vi "FRCts20_Backend_Comment_GET.vi"(6 "Message Attributes":T4, 8 "error in (no error)":errorcluster, 10 "Data":string, 11 "Engine_Refnums":T1) -> (0 "error out":errorcluster)   [LabVIEW 2014, in "FRCts20_Backend_Engine.lvlib"]
doc: "Retrieves all information about a comment, called by the Comment API. Expects a comment index."
uses:
  FRCts20_Backend_Engine.lvlib
  Dependencies/Keyed Array/KeyedArray.ctl
  FRCts20_Backend_EngineRefnums.ctl
  INI_Accessor/FRCts20_Backend_INI Controller.lvclass
  Dependencies/AMC/_SubVIs/TypeDefs/Message Queue.ctl
  Dependencies/AMC/_SubVIs/TypeDefs/Message.ctl
  <vilib>/addons/database/Connection.llb/Conn ObjectReference.ctl
  FRCts20_Backend_FGVOperation.ctl
  FRCts20_Backend_API/FRCts20_Backend_API_Note.ctl
  FRCts20_Backend_API/FRCts20_Backend_API.lvlib
  Dependencies/Keyed Array/Tools_KeyedArray.lvlib
  Dependencies/AMC/AMC.lvlib
  <vilib>/addons/database/NI_Database_API.lvlib
panel:
  # "DEPRICATED"
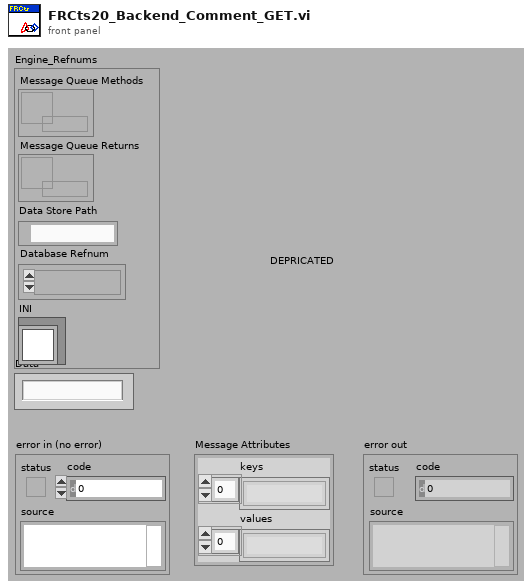
[diagram p1: front panel]
types:
  T1 = typedef "FRCts20_Backend_Engine.lvlib/FRCts20_Backend_EngineRefnums.ctl" = cluster{"Message Queue Methods":T2, "Message Queue Returns":T2, "Data Store Path":path, "Database Refnum":T3, "INI":refnum<class "FRCts20_Backend_INI Controller.lvclass">}
  T2 = typedef "AMC.lvlib/Message Queue.ctl" = refnum<queue>
  T3 = typedef "NI_Database_API.lvlib/Conn ObjectReference.ctl" = refnum<k1>
  T4 = typedef "Tools_KeyedArray.lvlib/KeyedArray.ctl" = cluster{"keys":string[], "values":string[]}
  T5 = typedef "FRCts20_Backend_Engine.lvlib/FRCts20_Backend_API.lvlib/FRCts20_Backend_API_Note.ctl" = cluster{"Note Index":u32, "Request Index":u32, "Author":string, "Time Entered":timestamp, "Text":string, "Solution":bool, "APIReturn":string}
  T6 = typedef "FRCts20_Backend_Engine.lvlib/FRCts20_Backend_FGVOperation.ctl" = enum16{"Initialize", "EnqueueMessage", "EnqueueDataReturn", "FlushMessage", "FlushDataReturn"}
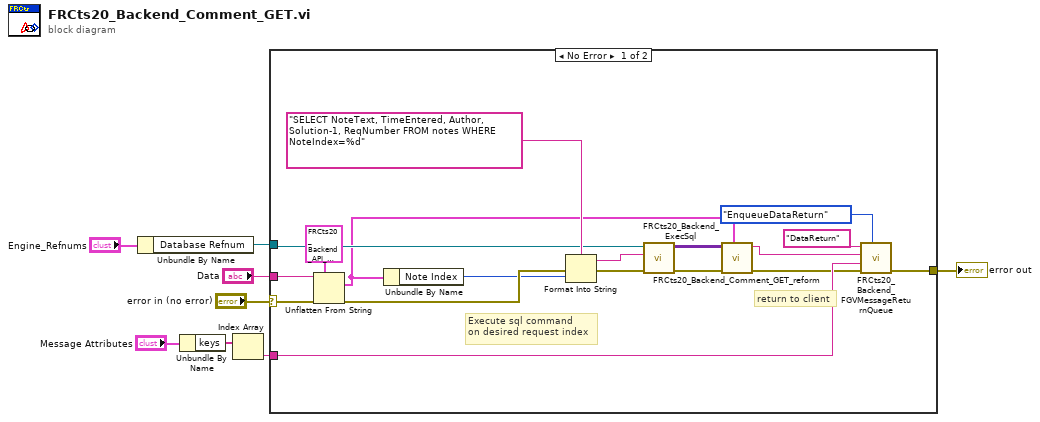
[diagram p0: block diagram]
diagram:
  n1 = Unbundle By Name("Engine_Refnums") -> ("Database Refnum"=w1:T3)
  n2 = Unbundle By Name("Message Attributes") -> ("keys"=w4:string[])
  n3 = Index Array(array=w4) -> (element=w3:string)  [unwired: 1 in]
  n4 = case shown="No Error" "error in (no error)" {
    selector: "error in (no error)" -> [w23 w27]
    tunnel: [w26 w27] -> w7
    tunnel: w1 -> [w14 _]
    tunnel: "Data" -> [w24 _]
    tunnel: w3 -> [w25 _]
    frame No Error {
      # "return to client"
      # "Execute sql command\non desired request index"
      n5 = Unflatten From String(type=T5 {"Note Index"=0, "Request Index"=0, "Author"="", "Time Entered"=timestamp(0 s since 1904-01-01), "Text"="", "Solution"=FALSE, "APIReturn"=""} ("Note"), binary string=w24, error in (no error)=w23) -> (value=w9:T5, error out=w22:errorcluster)  [unwired: 2 in, 1 out]
      n6 = Unbundle By Name(w9) -> ("Note Index"=w20:u32)
      n7 = Format Into String(format string="SELECT NoteText, TimeEntered, Author, Solution-1, ReqNumber FROM notes WHERE NoteIndex=%d", error in=w22, w20) -> (resulting string=w12:string, error out=w13:errorcluster)  [unwired: 1 in]
      n8 = call "FRCts20_Backend_ExecSql.vi"("error in (no error)"=w13, "format string"=w12, "Refnum in"=w14) -> ("error out"=w10:errorcluster, "recordset data"=w11:variant[][])  [unwired: 6 in, 1 out]
      n9 = call "FRCts20_Backend_Comment_GET_reform.vi"("Note"=w9, "error in (no error)"=w10, "recordset data"=w11) -> ("error out"=w16:errorcluster, "data string"=w17:string)  [unwired: 7 in]
      n10 = call "FRCts20_Backend_FGVMessageReturnQueue.vi"("Operation"=FRCts20_Backend_FGVOperation."EnqueueDataReturn", "error in (no error)"=w16, "Key"=w25, "Message Value"=w17, "Message Name"="DataReturn") -> ("error out"=w26:errorcluster)  [unwired: 5 in, 1 out]
    }
    frame Error {
    }
  }
  "error out" <- w7
